vi "ScaleFPS.vi"() -> ()   [LabVIEW 2019]
panel:
  in  "InitCluster.FPS":u16
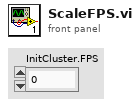
[diagram p1: front panel]
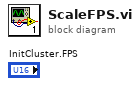
[diagram p0: block diagram]
diagram:
